vi "SEND ADC.vi"(8 "error in (no error)":errorcluster, 10 "CANAL":u8, 11 "SERIAL DEVICE in":refnum<class "SERIAL DEVICE.lvclass">) -> (0 "error out":errorcluster, 2 "read buffer":string, 3 "SERIAL DEVICE out":refnum<class "SERIAL DEVICE.lvclass">)   [LabVIEW 2019, in "SERIAL DEVICE.lvclass"]
uses:
  SERIAL DEVICE.lvclass
  SERIAL DEVICE.lvclass/SERIAL DEVICE.ctl
  9f88877d-c6d6-43aa-9861-71a693b3c7d2.vi
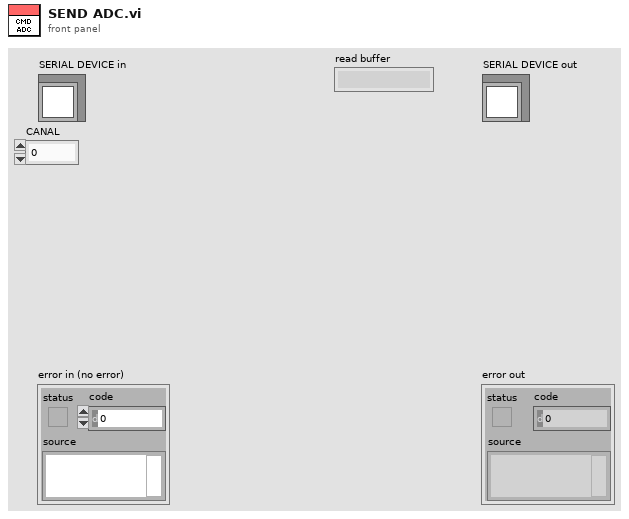
[diagram p1: front panel]
types:
  T1 = typedef "MICROS.ctl" = string
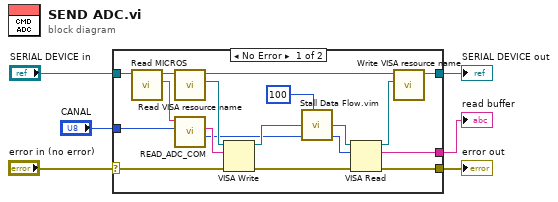
[diagram p0: block diagram]
diagram:
  n1 = case shown="No Error" "error in (no error)" {
    selector: "error in (no error)" -> [w10 w25]
    tunnel: [w9 w25] -> w5
    tunnel: [w12 w24] -> w3
    tunnel: "SERIAL DEVICE in" -> [w23 w24]
    tunnel: "CANAL" -> [w21 _]
    tunnel: [w15 _] -> w1
    frame No Error {
      n2 = call "Read MICROS.vi"("SERIAL DEVICE in"=w23) -> ("MICROS"=w22:T1, "SERIAL DEVICE out"=w8:refnum<class "SERIAL DEVICE.lvclass">)  [unwired: 8 in, 1 out]
      n3 = call "Read VISA resource name.vi"("SERIAL DEVICE in"=w8) -> ("VISA resource name"=w20:refnum<visa-resource-name>, "SERIAL DEVICE out"=w13:refnum<class "SERIAL DEVICE.lvclass">)  [unwired: 8 in, 1 out]
      n4 = call "READ_ADC_COM.vi"("CANAL"=w21, "MICROS"=w22) -> ("BYTES EXPECTED"=w16:i32, "COMANDO"=w19:string)  [unwired: 7 in, 1 out]
      n5 = VISA Write(VISA resource name=w20, write buffer=w19, error in (no error)=w10) -> (VISA resource name out=w18:refnum<visa-resource-name>, error out=w11:errorcluster)  [unwired: 1 out]
      n6 = call "Stall Data Flow.vim"("value in"=w18, "milliseconds to wait"=u32 100) -> ("value out"=w17:refnum<visa-resource-name>)  [unwired: 1 out]
      n7 = VISA Read(VISA resource name=w17, byte count=w16, error in (no error)=w11) -> (VISA resource name out=w14:refnum<visa-resource-name>, read buffer=w15:string, error out=w9:errorcluster)  [unwired: 1 out]
      n8 = call "Write VISA resource name.vi"("VISA resource name"=w14, "SERIAL DEVICE in"=w13) -> ("SERIAL DEVICE out"=w12:refnum<class "SERIAL DEVICE.lvclass">)  [unwired: 8 in, 1 out]
    }
    frame Error {
    }
  }
  "error out" <- w5
  "SERIAL DEVICE out" <- w3
  "read buffer" <- w1
